vi "Waveform.vi"(5 "signal type":string) -> (2 "signal type":T1(ring))   [LabVIEW 2016]
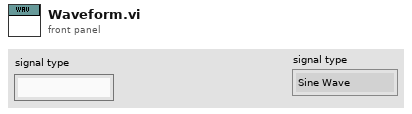
[diagram p1: front panel]
types:
  T1 = enum16{"Sine Wave", "Triangle Wave", "Square Wave", "Sawtooth Wave"}
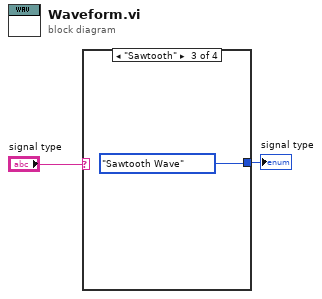
[diagram p0: block diagram]
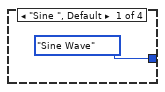
[diagram p2: hidden frame]
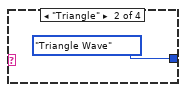
[diagram p3: hidden frame]
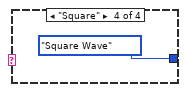
[diagram p4: hidden frame]
diagram:
  n1 = case shown="\"Sawtooth\"" "signal type" {
    tunnel: [T1."Sine Wave" ("signal type") T1."Triangle Wave" ("signal type") T1."Sawtooth Wave" ("signal type") T1."Square Wave" ("signal type")] -> w1
    frame "Sine ", Default {
    }
    frame "Triangle" {
    }
    frame "Sawtooth" {
    }
    frame "Square" {
    }
  }
  "signal type" <- w1
